vi "Sensor information.vi"(8 "error in (no error)":errorcluster, 10 "Table":string[][](table)) -> (0 "error in (no error) 2":errorcluster)   [LabVIEW 2015]
uses:
  Control Button/Exit.ctl
  Control Button/Save.ctl
  <vilib>/Utility/miscctls.llb/LVRowAndColumnTypeDef.ctl
panel:
  in  "stop":T1
  in  "Save Button":T2
  out "Active Cell:Active Cell":T3
  # "Sensor Information"
  # "Sensor Name & Unit"
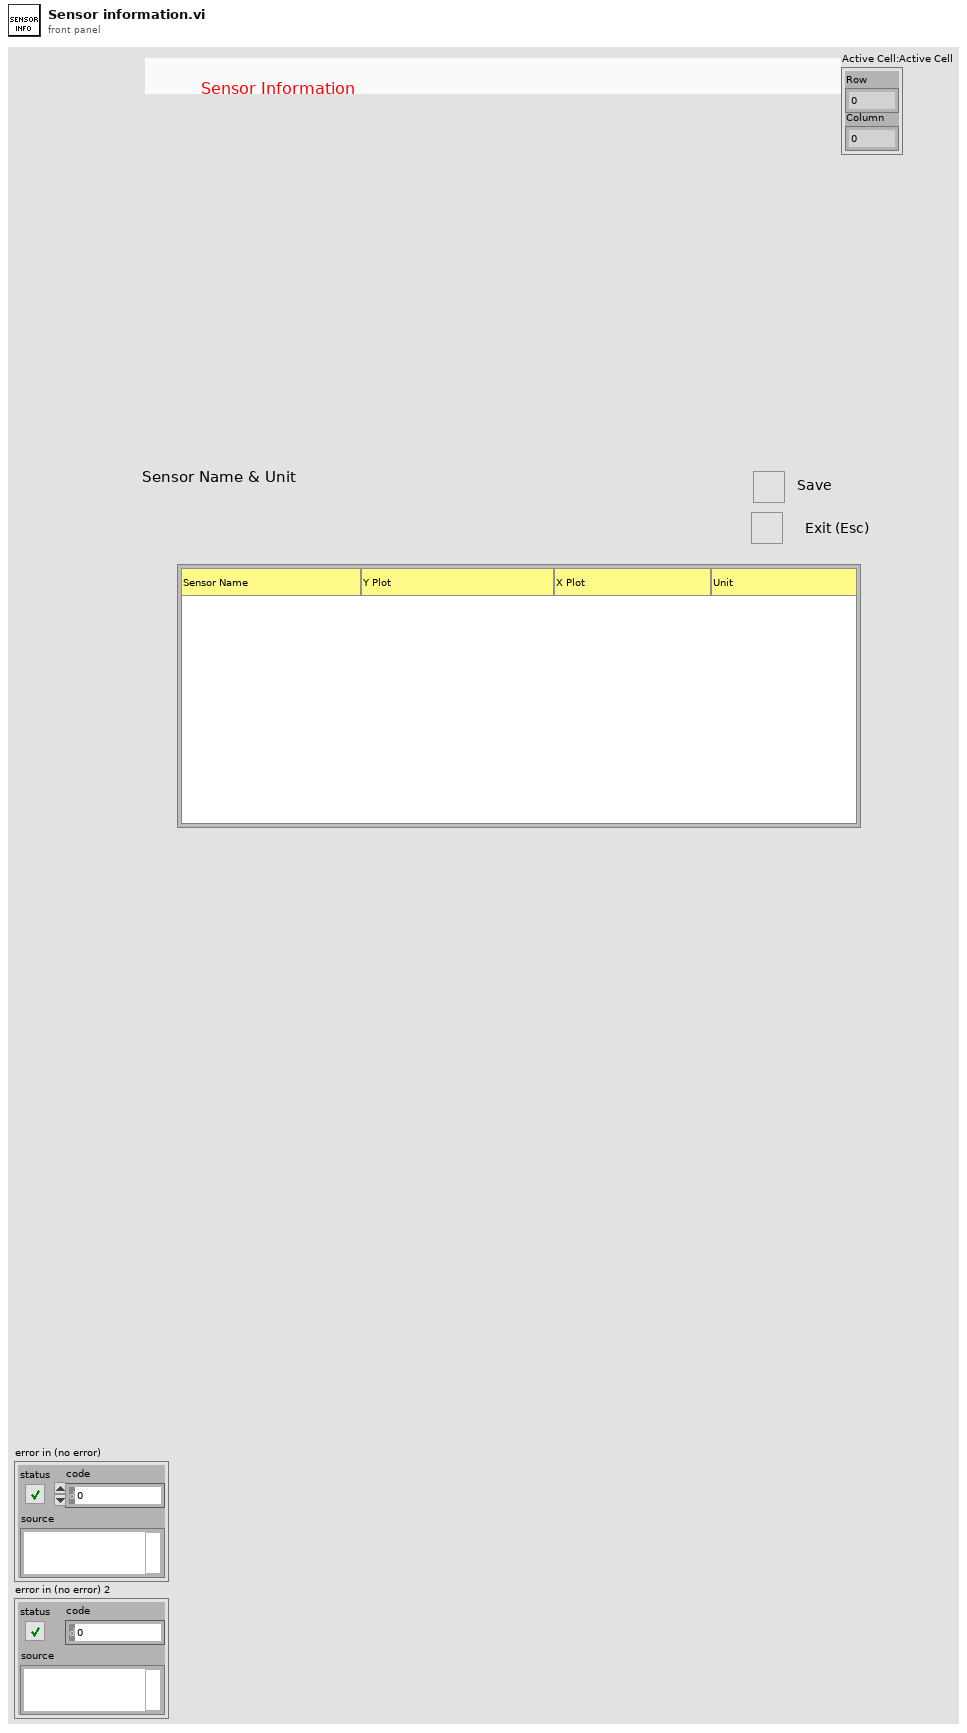
[diagram p1: front panel]
types:
  T1 = typedef "Exit.ctl" = bool
  T2 = typedef "Save.ctl" = bool
  T3 = typedef "LVRowAndColumnTypeDef.ctl" = cluster{"Row":i32, "Column":i32}
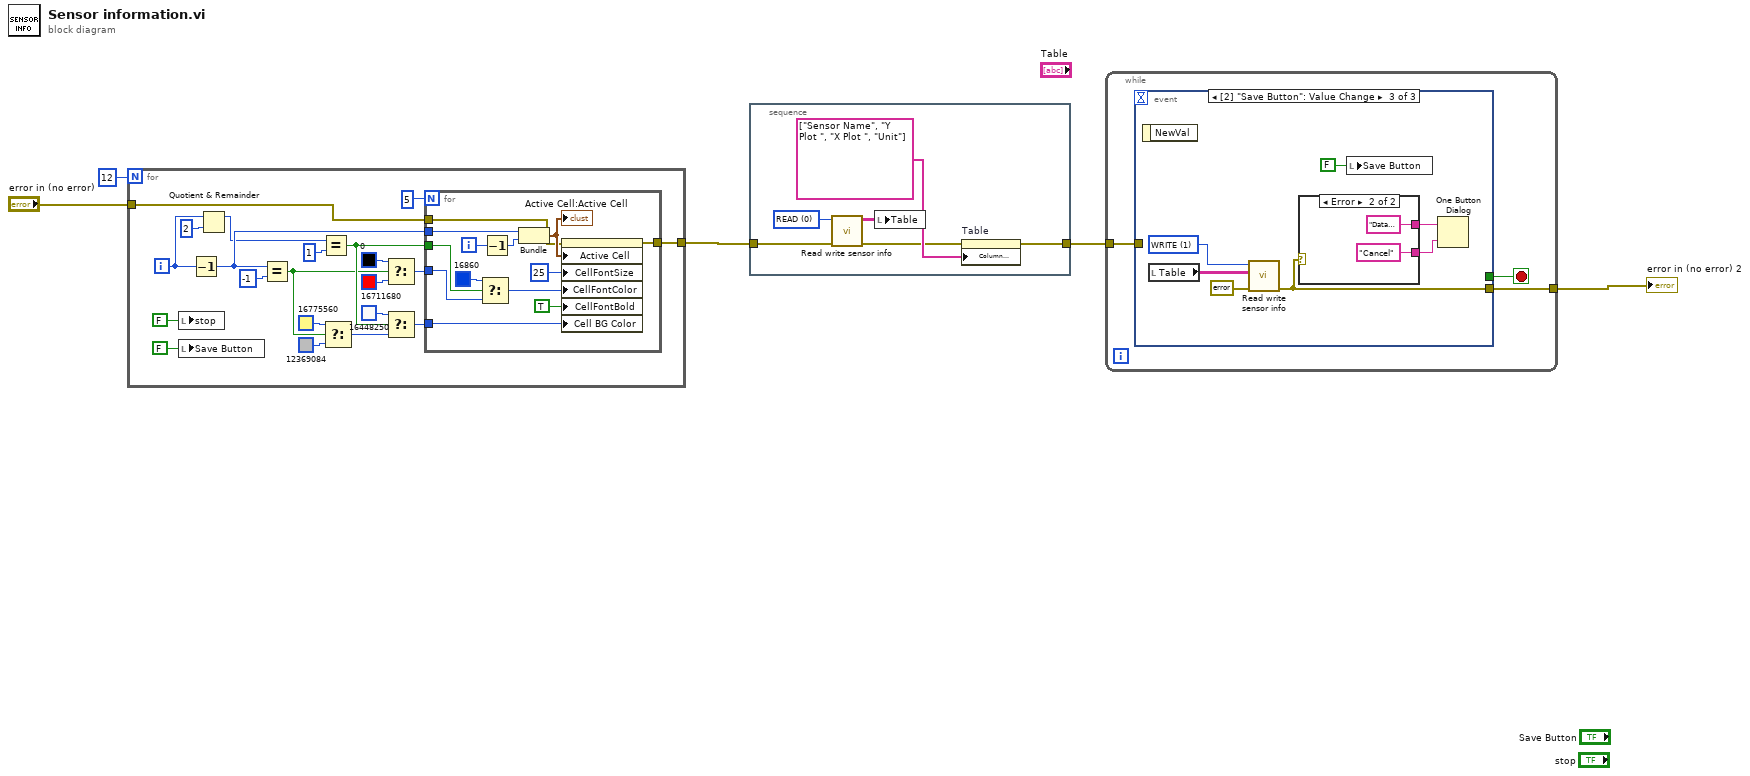
[diagram p0: block diagram]
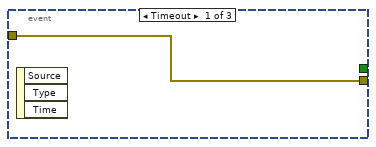
[diagram p2: hidden frame]
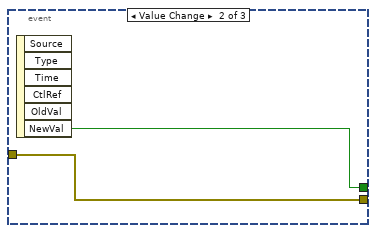
[diagram p3: hidden frame]
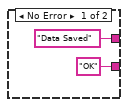
[diagram p4: hidden frame]
diagram:
  n1 = for {
    N: 12 -> [_]
    tunnel: [w9] -> w2
    tunnel: "error in (no error)" -> [w8]
    i -> [w21]
    n2 = local write "stop"(FALSE ("stop")) -> ()
    n3 = local write "Save Button"(FALSE ("Save Button")) -> ()
    n4 = Decrement(x=w21) -> (x-1=w19:i32)
    n5 = Quotient & Remainder(x=w21, y=2) -> (x-y*floor(x/y)=w15:i32)  [unwired: 1 out]
    n6 = Equal?(x=w19, y=-1) -> (x = y?=w12:bool)
    n7 = Equal?(x=w15, y=1) -> (x = y?=w14:bool)
    n8 = Select(t=u32 16775560 ("Color Box"), s=w12, f=u32 12369084 ("Color Box")) -> (s? t:f=w16:u32)
    n9 = Select(t=u32 0 ("Color Box"), s=w12, f=u32 16711680 ("Color Box")) -> (s? t:f=w10:u32)
    n10 = Select(t=u32 16448250 ("Color Box"), s=w14, f=w16) -> (s? t:f=w22:u32)
    n11 = for {
      N: 5 -> [_]
      tunnel: w22 -> [w34]
      tunnel: w19 -> [w38]
      tunnel: w14 -> [w31]
      tunnel: w10 -> [w30]
      tunnel: [w28] -> w9
      tunnel: w8 -> [w27]
      i -> [w37]
      n12 = Select(t=u32 16860 ("Color Box"), s=w31, f=w30) -> (s? t:f=w29:u32)
      n13 = Decrement(x=w37) -> (x-1=w33:i32)
      n14 = Bundle(w38, w33) -> (w36:cluster{i32, i32})  [unwired: 1 in]
      "Active Cell:Active Cell" <- w36
      n15 = property on="Table" class="Tbl (strict)"(error in=w27, "Active Cell"=w36, "CellFontSize"=u32 25 ("Active Cell:Cell Font:Size"), "CellFontColor"=w29, "CellFontBold"=TRUE ("Active Cell:Cell Font:Bold"), "Cell BG Color"=w34) -> (error out=w28:errorcluster)  [unwired: 1 in, 1 out]
    }
  }
  n16 = stacked-sequence {
    tunnel: [w44] -> w5
    tunnel: w2 -> [w41]
    frame #0 {
      w43 = u16 0 items=["READ", "WRITE"] ("Read/Write")
      n17 = call "Read write sensor info.vi"("error in (no error)"=w41, "Read/Write"=w43) -> ("error out"=w40:errorcluster, "Table Control out"=w42:string[][])  [unwired: 8 in]
      n18 = local write "Table"(w42) -> ()
      n19 = property on="Table" class="Tbl (strict)"(error in=w40, "Column Headers[]"=string[] ["Sensor Name", "Y Plot ", "X Plot ", "Unit"] ("Table Control")) -> (error out=w44:errorcluster)  [unwired: 1 in, 1 out]
    }
  }
  n20 = while {
    tunnel: w5 -> [w48]
    tunnel: [w47] -> w4
    stop <- w46 stop-if-true
    n21 = event shown="[2] \"Save Button\": Value Change" {
      selector: _ -> [_ _ _]
      dyn-events: _ -> [_ _ _]
      timeout: _ -> [_ _ _]
      tunnel: w48 -> [w49 w50 _]
      tunnel: [w49 w50 w55] -> w47
      tunnel: [_ w51 _] -> w46
      event Timeout {
        n22 = event-data() -> ()  [unwired: 1 in, 3 out]
      }
      event Value Change {
        n23 = event-data() -> ("NewVal"=w51:T1)  [unwired: 1 in, 5 out]
      }
      event Value Change {
        w58 = u16 1 items=["READ", "WRITE"] ("Read/Write")
        n24 = event-data() -> ()  [unwired: 1 in, 1 out]
        n25 = local read "Table"() -> (w52:string[][])
        n26 = call "Read write sensor info.vi"("error in (no error)"=errorcluster {"status"=FALSE, "code"=0, "source"=""}, "Table Control in"=w52, "Read/Write"=w58) -> ("error out"=w55:errorcluster)  [unwired: 7 in, 1 out]
        n27 = case shown="Error" w55 {
          tunnel: ["Data Saved" ("message") "Data Not Saved,Check The File Path" ("message")] -> w54
          tunnel: ["OK" ("button name (\"OK\")") "Cancel" ("button name (\"OK\")")] -> w53
          frame No Error {
          }
          frame Error {
          }
        }
        n28 = local write "Save Button"(FALSE ("Save Button")) -> ()
        n29 = One Button Dialog(message=w54, button name ("OK")=w53) -> ()  [unwired: 1 out]
      }
    }
  }
  "error in (no error) 2" <- w4
